vi "DB_Insert_Block_Report.vi"(0 "Numeric (DATO)":i8=-77, 2 "date/time string":string, 5 "Numeric (DATO) 2":i8=-77, 7 "BIT (DATO)":i32=1203, 9 "BIT (DATO) 2":i32=1203, 11 "Numeric (DATO) 3":i8=-77) -> ()   [LabVIEW 2017]
uses:
  <vilib>/addons/database/Connection.llb/DB Tools Open Connec (String).vi
  <vilib>/addons/database/NI_Database_API.lvlib
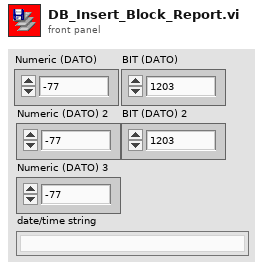
[diagram p1: front panel]
types:
  T1 = typedef "NI_Database_API.lvlib/Conn ObjectReference.ctl" = refnum<k1>
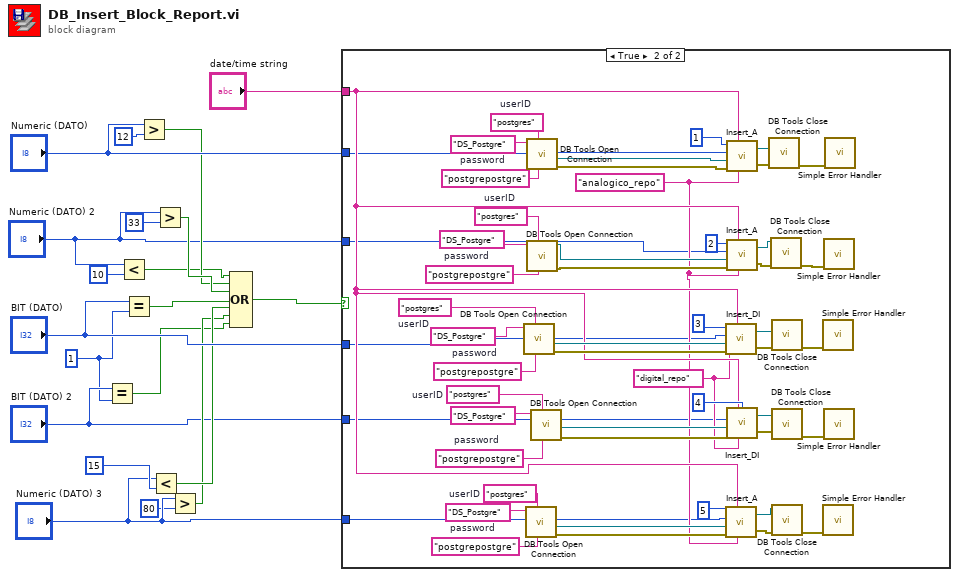
[diagram p0: block diagram]
diagram:
  w5 = 1 ("y")
  n1 = Equal?(x="BIT (DATO) 2", y=w5) -> (x = y?=w4:bool)
  n2 = Less?(x="Numeric (DATO) 2", y=i8 10) -> (x < y?=w1:bool)
  n3 = Equal?(x="BIT (DATO)", y=w5) -> (x = y?=w18:bool)
  n4 = Greater?(x="Numeric (DATO)", y=i8 12) -> (0:w12:bool)
  n5 = Less?(x="Numeric (DATO) 3", y=i8 15) -> (x < y?=w10:bool)
  n6 = Greater?(x="Numeric (DATO) 2", y=i8 33) -> (0:w15:bool)
  n7 = Greater?(x="Numeric (DATO) 3", y=i8 80) -> (0:w7:bool)
  n8 = Compound Arithmetic op=OR(w1, w12, w15, w18, w10, w7, w4) -> (w17:bool)
  n9 = case shown="True" w17 {
    tunnel: "date/time string" -> [_ w28]
    tunnel: "Numeric (DATO)" -> [_ w25]
    tunnel: "Numeric (DATO) 2" -> [_ w24]
    tunnel: "BIT (DATO)" -> [_ w23]
    tunnel: "BIT (DATO) 2" -> [_ w22]
    tunnel: "Numeric (DATO) 3" -> [_ w21]
    frame False {
    }
    frame True {
      w26 = "digital_repo" ("table")
      w27 = "analogico_repo" ("table")
      w41 = "postgrepostgre"  # password
      w43 = "postgres"  # userID
      w44 = "postgrepostgre"  # password
      w46 = "postgres"  # userID
      w51 = "postgrepostgre"  # password
      w53 = "postgres"  # userID
      w54 = "postgrepostgre"  # password
      w56 = "postgres"  # userID
      w57 = "postgrepostgre"  # password
      w59 = "postgres"  # userID
      n10 = call-poly <vilib>:"DB Tools Open Connection.vi"("password"=w41, "userID"=w43, "connection information"="DS_Postgre") -> ("error out"=w39:errorcluster, "connection reference"=w40:T1)  [unwired: 5 in]
      n11 = call-poly <vilib>:"DB Tools Open Connection.vi"("password"=w54, "userID"=w56, "connection information"="DS_Postgre") -> ("error out"=w49:errorcluster, "connection reference"=w50:T1)  [unwired: 5 in]
      n12 = call-poly <vilib>:"DB Tools Open Connection.vi"("password"=w57, "userID"=w59, "connection information"="DS_Postgre") -> ("error out"=w34:errorcluster, "connection reference"=w35:T1)  [unwired: 5 in]
      n13 = call-poly <vilib>:"DB Tools Open Connection.vi"("password"=w44, "userID"=w46, "connection information"="DS_Postgre") -> ("error out"=w31:errorcluster, "connection reference"=w30:T1)  [unwired: 5 in]
      n14 = call-poly <vilib>:"DB Tools Open Connection.vi"("password"=w51, "userID"=w53, "connection information"="DS_Postgre") -> ("error out"=w47:errorcluster, "connection reference"=w48:T1)  [unwired: 5 in]
      n15 = call "Insert_DI.vi"("table"=w26, "date/time string"=w28, "error in (no error)"=w39, "connection reference"=w40, "BIT (DATO)"=w23, "Numeric (ID_SENSOR)"=3) -> ("error out"=w64:errorcluster, "connection reference out"=w65:T1)
      n16 = call "Insert_A.vi"("table"=w27, "date/time string"=w28, "error in (no error)"=w49, "connection reference"=w50, "Numeric (DATO)"=w21, "Numeric (ID_SENSOR)"=5) -> ("error out"=w60:errorcluster, "connection reference out"=w61:T1)
      n17 = call "Insert_A.vi"("table"=w27, "date/time string"=w28, "error in (no error)"=w34, "connection reference"=w35, "Numeric (DATO)"=w25, "Numeric (ID_SENSOR)"=1) -> ("error out"=w37:errorcluster, "connection reference out"=w38:T1)
      n18 = call "Insert_A.vi"("table"=w27, "date/time string"=w28, "error in (no error)"=w31, "connection reference"=w30, "Numeric (DATO)"=w24, "Numeric (ID_SENSOR)"=2) -> ("error out"=w32:errorcluster, "connection reference out"=w33:T1)
      n19 = call "Insert_DI.vi"("table"=w26, "date/time string"=w28, "error in (no error)"=w47, "connection reference"=w48, "BIT (DATO)"=w22, "Numeric (ID_SENSOR)"=4) -> ("error out"=w62:errorcluster, "connection reference out"=w63:T1)
      n20 = call <vilib>:"DB Tools Close Connection.vi"("error in (no error)"=w37, "connection reference"=w38) -> ("error out"=w70:errorcluster)  [unwired: 5 in]
      n21 = call <vilib>:"DB Tools Close Connection.vi"("error in (no error)"=w32, "connection reference"=w33) -> ("error out"=w69:errorcluster)  [unwired: 5 in]
      n22 = call <vilib>:"DB Tools Close Connection.vi"("error in (no error)"=w64, "connection reference"=w65) -> ("error out"=w68:errorcluster)  [unwired: 5 in]
      n23 = call <vilib>:"DB Tools Close Connection.vi"("error in (no error)"=w62, "connection reference"=w63) -> ("error out"=w67:errorcluster)  [unwired: 5 in]
      n24 = call <vilib>:"DB Tools Close Connection.vi"("error in (no error)"=w60, "connection reference"=w61) -> ("error out"=w66:errorcluster)  [unwired: 5 in]
      n25 = call <vilib>:"Simple Error Handler.vi"("error in (no error)"=w68) -> ()  [unwired: 4 in, 5 out]
      n26 = call <vilib>:"Simple Error Handler.vi"("error in (no error)"=w66) -> ()  [unwired: 4 in, 5 out]
      n27 = call <vilib>:"Simple Error Handler.vi"("error in (no error)"=w69) -> ()  [unwired: 4 in, 5 out]
      n28 = call <vilib>:"Simple Error Handler.vi"("error in (no error)"=w67) -> ()  [unwired: 4 in, 5 out]
      n29 = call <vilib>:"Simple Error Handler.vi"("error in (no error)"=w70) -> ()  [unwired: 4 in, 5 out]
    }
  }
